vi "Update bitfile.vi"(8 "error in (no error)":errorcluster, 9 "FPGA addon name":string="FPGA Addon", 10 "bitfile name":string="TestBitfile2.lvbitx", 11 "sysdef path in":path) -> (0 "error out":errorcluster, 3 "sysdef path out":path)   [LabVIEW 2018, in "Bitfile Reload System Tests.lvclass"]
uses:
  Bitfile Reload System Tests.lvclass
  APIs/Scripting API/Scripting API.lvlib
  Addon/Addon System Explorer/FPGA Addon System Explorer.lvlib
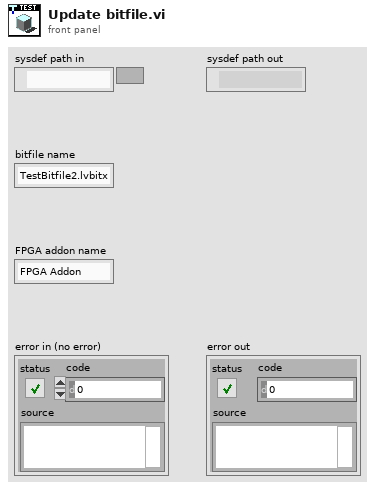
[diagram p1: front panel]
types:
  T1 = typedef "Custom Device API.lvlib/Custom Device Item Ref.ctl" = u64
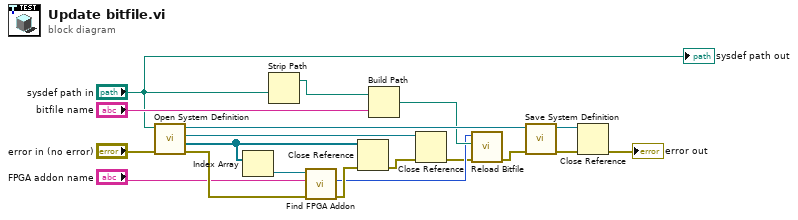
[diagram p0: block diagram]
diagram:
  n1 = call "Open System Definition.vi"("error in (no error)"="error in (no error)", "System Definition File"="sysdef path in") -> ("error out"=w9:errorcluster, "targets refnums"=w16:refnum<k24>[], "root refnum"=w2:refnum<k24>, "system definition refnum"=w13:refnum<k24>)  [unwired: 6 in]
  n2 = Index Array(array=w16) -> (element=w8:refnum<k24>)  [unwired: 1 in]
  n3 = Strip Path(path="sysdef path in") -> (stripped path=w4:path)  [unwired: 1 out]
  n4 = call "Find FPGA Addon.vi"("error in"=w9, "FPGA addon name"="FPGA addon name", "target in"=w8) -> ("error out"=w15:errorcluster, "FPGA addon refnum out"=w6:T1)  [unwired: 5 in, 2 out]
  n5 = Close Reference(reference=w16, error in (no error)=w15) -> (error out=w3:errorcluster)
  n6 = Build Path(base path=w4, name or relative path="bitfile name") -> (appended path=w11:path)
  n7 = Close Reference(reference=w2, error in (no error)=w3) -> (error out=w1:errorcluster)
  n8 = call "Reload Bitfile.vi"("error in (no error)"=w1, "NewVal"=w11, "Item Ref in"=w6) -> ("error out"=w12:errorcluster)  [unwired: 7 in, 1 out]
  n9 = call "Save System Definition.vi"("error in (no error)"=w12, ".NET Refnum in"=w13) -> ("error out"=w17:errorcluster, ".NET Refnum out"=w18:refnum<k24>)  [unwired: 8 in]
  n10 = Close Reference(reference=w18, error in (no error)=w17) -> (error out=→"error out":errorcluster)
  "sysdef path out" <- "sysdef path in"
